vi "Lucid for Paul.vi"() -> ()   [LabVIEW 2020]
uses:
  338aad08-1463-4498-a797-5b4852814611.vi
  4138bf18-c343-47f1-a243-b6a61443ea43.vi
  <vilib>/JDP Science/JSONtext/JSONtext.lvlib
panel:
  in  "system_data":T1
  out "Array 2":T2(array[cluster])
  in  "string_data":string
  in  "Array":T2(array[cluster])
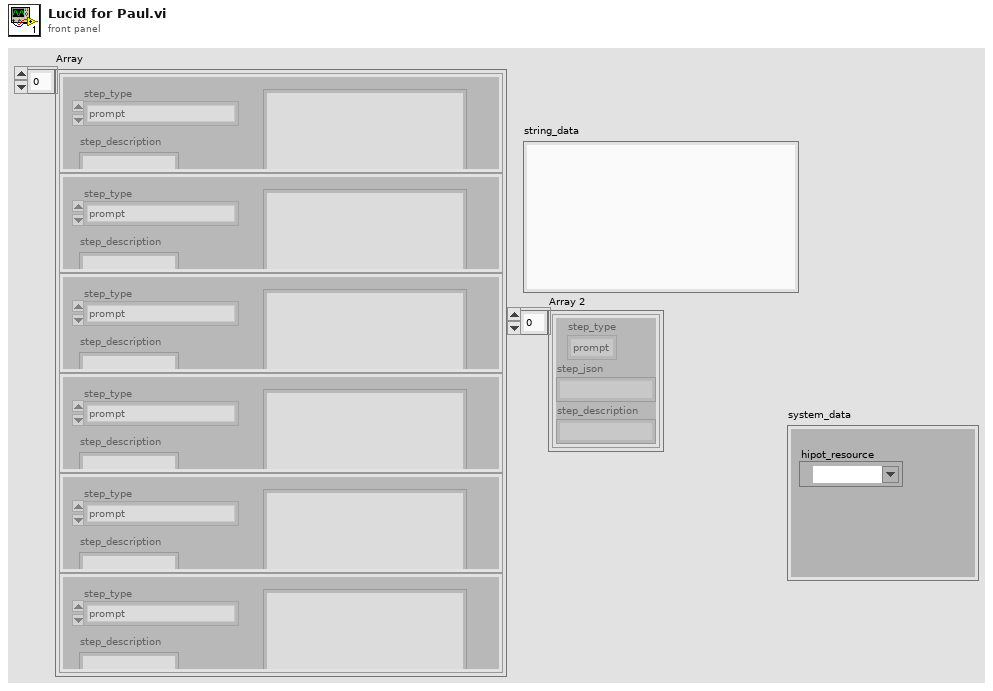
[diagram p1: front panel]
types:
  T1 = cluster{"hipot_resource":refnum<visa-resource-name>}
  T2 = cluster{"step_type":enum16{"prompt", "send sequence #", "hi-pot on"}, "step_json":string, "step_description":string}[]
  T3 = cluster{"step_type":enum16{"prompt", "send sequence #", "hi-pot on"}, "step_json":string}
  T4 = cluster{"step_type":enum16{"prompt", "send sequence #", "hi-pot on"}, "step_json":string, "step_description":string}
  T5 = cluster{"step_description":string, "step_type":enum16{"prompt", "send sequence #", "hi-pot on"}}
  T6 = cluster{i32, "Cluster":cluster{"step_type":enum16{"prompt", "send sequence #", "hi-pot on"}, "step_json":string}, "session_ref":i32, "system_data":cluster{"hipot_resource":refnum<visa-resource-name>}, "error constant":errorcluster, "results":i32}
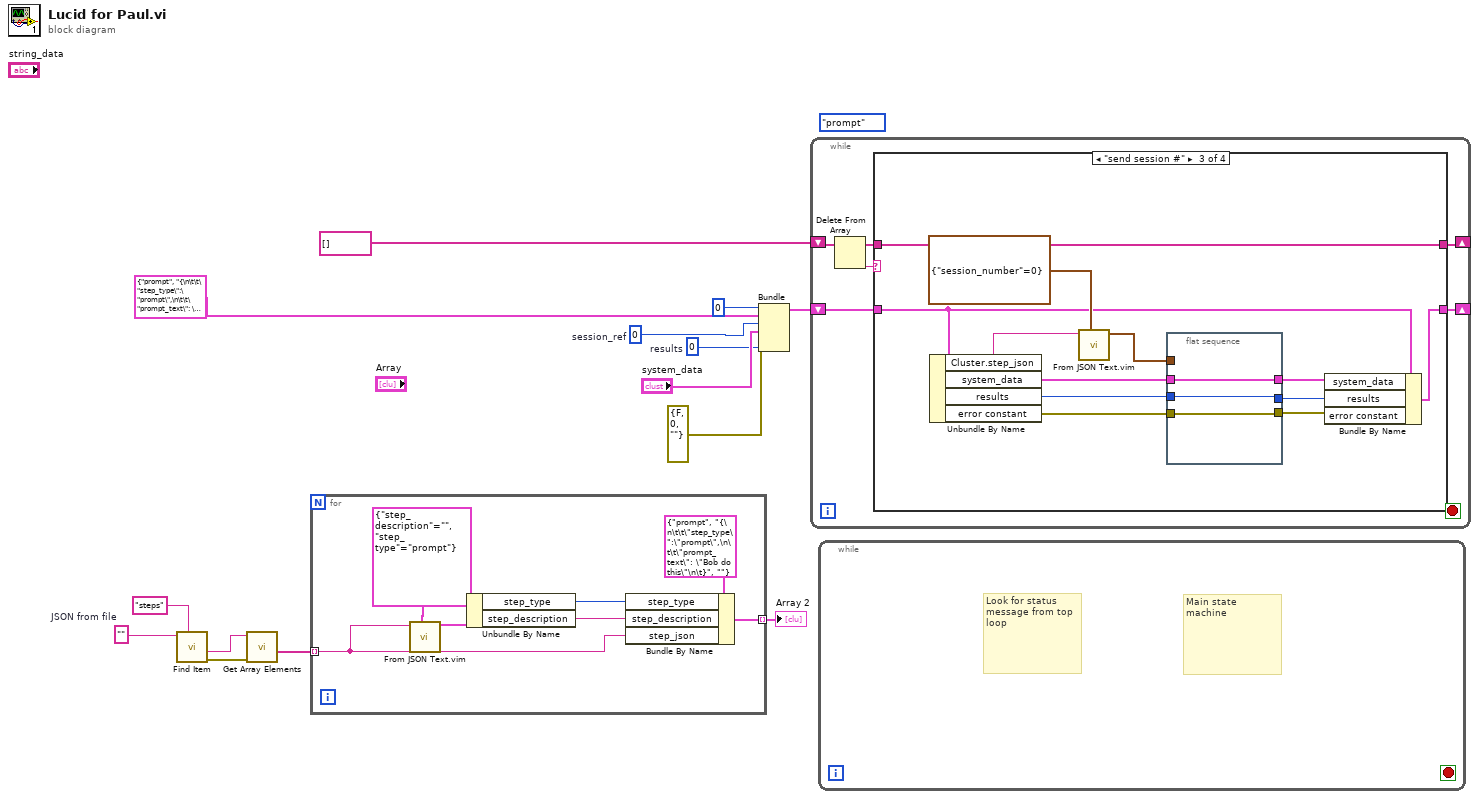
[diagram p0: block diagram]
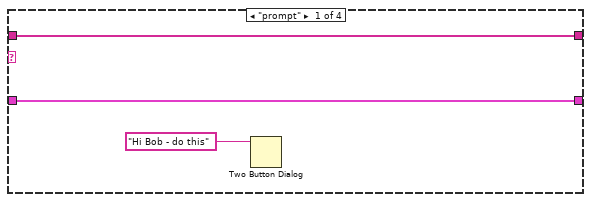
[diagram p2: hidden frame]
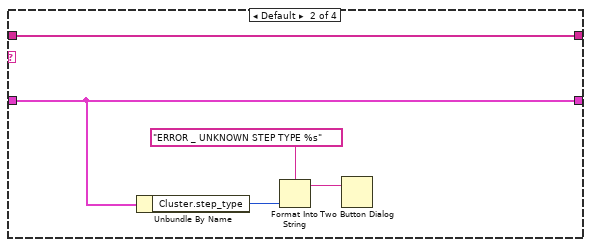
[diagram p3: hidden frame]
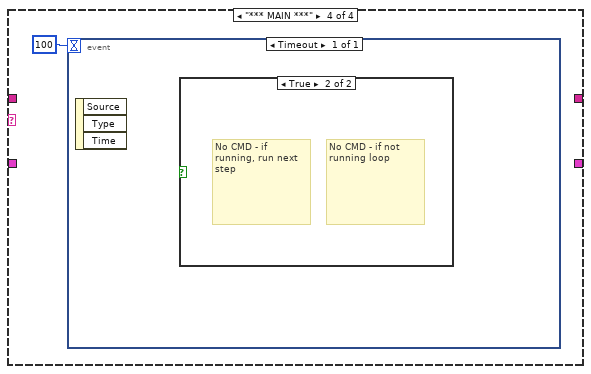
[diagram p4: hidden frame]
diagram:
  w1 = 0  # results
  w4 = 0  # session_ref
  (unwired) enum16{"prompt", "send sequence #", "hi-pot on"}."prompt" ("step_type")
  w9 = ""  # JSON from file
  n1 = call <vilib>:"Find Item.vi"("$Path or Item Name"="steps", "JSON"=w9) -> ("error out"=w8:errorcluster, "<JSON>"=w7:string)  [unwired: 6 in, 2 out]
  n2 = call <vilib>:"Get Array Elements.vi"("error in (no error)"=w8, "JSON"=w7) -> ("<JSON>"=w6:string[])  [unwired: 7 in, 2 out]
  n3 = for {
    tunnel: w6 -> [w16] mode=indexing
    tunnel: [w15] -> w5 mode=indexing
    n4 = call "From JSON Text.vim"("Data Type and Default Value"=T5 {"step_description"="", "step_type"=enum."prompt"}, "JSON"=w16) -> ("Data out"=w19:T5)  [unwired: 8 in, 1 out]
    n5 = Unbundle By Name(w19) -> ("step_type"=w18:enum16{"prompt", "send sequence #", "hi-pot on"}, "step_description"=w17:string)
    n6 = Bundle By Name(cluster=T4 {"step_type"=enum."prompt", "step_json"="{\n\t\t\"step_type\":\"prompt\",\n\t\t\"prompt_text\": \"Bob do this\"\n\t}", "step_description"=""} ("Cluster"), "step_type"=w18, "step_description"=w17, "step_json"=w16) -> (w15:T4)
  }
  "Array 2" <- w5
  n7 = Bundle(0, "Cluster"=T3 {"step_type"=enum."prompt", "step_json"="{\n\t\t\"step_type\":\"prompt\",\n\t\t\"prompt_text\": \"Bob do this\"\n\t}"}, "session_ref"=w4, "system_data"="system_data", "error constant"=errorcluster {"status"=FALSE, "code"=0, "source"=""}, "results"=w1) -> (w12:T6)  [unwired: 1 in]
  n8 = while {
    shift-right: [w24] -> _
    shift-left: string[] [] -> [w27]
    shift-right: [w22] -> _
    shift-left: w12 -> [w23]
    stop <- _ stop-if-true
    n9 = Delete From Array(array=w27) -> (deleted portion=w26:string, array with subset deleted=w25:string[])  [unwired: 2 in]
    n10 = case shown="\"send session #\"" w26 {
      tunnel: w25 -> [w29 w35 w47 _]
      tunnel: [w29 w35 w47 _] -> w24
      tunnel: w23 -> [w28 w34 w40 _]
      tunnel: [w28 w34 w41 _] -> w22
      frame "prompt" {
        n11 = Two Button Dialog(message="Hi Bob - do this") -> ()  [unwired: 2 in, 1 out]
      }
      frame Default {
        n12 = Unbundle By Name(w34) -> ("Cluster.step_type"=w33:enum16{"prompt", "send sequence #", "hi-pot on"})
        n13 = Format Into String(format string="ERROR _ UNKNOWN STEP TYPE %s" ("message"), w33) -> (resulting string=w31:string)  [unwired: 2 in, 1 out]
        n14 = Two Button Dialog(message=w31) -> ()  [unwired: 2 in, 1 out]
      }
      frame "send session #" {
        n15 = Unbundle By Name(w40) -> ("Cluster.step_json"=w46:string, "system_data"=w44:T1, "results"=w38:i32, "error constant"=w36:errorcluster)
        n16 = call "From JSON Text.vim"("Data Type and Default Value"=cluster{"session_number":i32} {"session_number"=0}, "JSON"=w46) -> ("Data out"=w43:cluster{"session_number":i32})  [unwired: 8 in, 1 out]
        n17 = flat-sequence {
          tunnel: w44 -> [w50]
          tunnel: w43 -> [_]
          tunnel: [w50] -> w42
          tunnel: [w48] -> w39
          tunnel: w38 -> [w49]
          tunnel: [w49] -> w37
          tunnel: w36 -> [w48]
          frame #0 {
          }
        }
        n18 = Bundle By Name(cluster=w40, "system_data"=w42, "results"=w37, "error constant"=w39) -> (w41:T6)
      }
      frame "*** MAIN ***" {
        n19 = event shown="[0] Timeout" {
          selector: _ -> [_]
          dyn-events: _ -> [_]
          timeout: 100 -> [_]
          event Timeout {
            n20 = event-data() -> ()  [unwired: 1 in, 3 out]
            n21 = case shown="True" {
              selector: _ -> [_ _]
              frame False {
              }
              frame True {
                # "No CMD - if not running loop"
                # "No CMD - if running, run next step"
              }
            }
          }
        }
      }
    }
  }
  n22 = while {
    stop <- _ stop-if-true
    # "Look for status message from top loop"
    # "Main state machine"
  }
